vi "testtest.vi"() -> ()   [LabVIEW 2019]
uses:
  <vilib>/WPC Systems Ltd/GECO Driver/Lib/GECOBase/GECO_Driver Class/GECO_SlotName.ctl
  <vilib>/WPC Systems Ltd/GECO Driver/GECODriver/GECO_Initialize_RT/Initialize VIs/Initialize_GECOUnoRT_4HX.vi
  <vilib>/WPC Systems Ltd/GECO Driver/Lib/GECOBase/GECO_Driver Class/Motion/_typedefine/GECO_Motion Operation Mode.ctl
  <vilib>/WPC Systems Ltd/GECO Driver/Lib/GECOBase/GECO_Driver Class/GECO_Driver.lvclass
  <vilib>/WPC Systems Ltd/GECO Driver/Lib/GECOBase/GECO_Driver Class/Motion/_typedefine/GECO_ActiveHighLow.ctl
panel:
  in  "Stop Move":bool
  out "Move Complete?":bool
  out "Logical Position":i32
  out "Encoder Position":i32
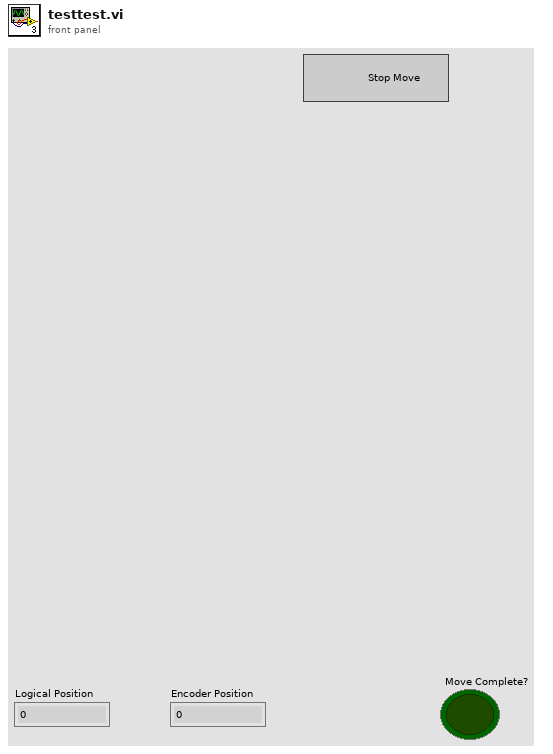
[diagram p1: front panel]
types:
  T1 = typedef "GECO_Driver.lvclass/GECO_SlotName.ctl" = enum16{"C1", "C2", "C3", "C4"}
  T2 = typedef "GECO_Driver.lvclass/GECO_ActiveHighLow.ctl" = enum16{"Active High", "Active Low"}
  T3 = cluster{"Forward Enable":bool, "Forward Polarity":T2}
  T4 = cluster{"Reverse Enable":bool, "Reverse Polarity":T2}
  T5 = typedef "GECO_Driver.lvclass/GECO_Motion Operation Mode.ctl" = enum16{"Absolute Position", "Relative Position", "Velocity"}
  T6 = cluster{"Motion Operation Mode":T5, "Target Position (0)":i32, "Velocity (10000)":i32, "Acceleration (100000)":u32, "Deacceleration (100000)":u32}
  T7 = enum16{"Step/Dir(One Pulse)", "CW/CCW(Two Pulse)"}
  T8 = enum16{"Absolute Position", "Relative Position", "Velocity"}
  T9 = typedef "GECO Motion.lvclass/Axis Select.ctl" = enum16{"Axis 1", "Axis 2", "Axis 3", "Axis 4"}
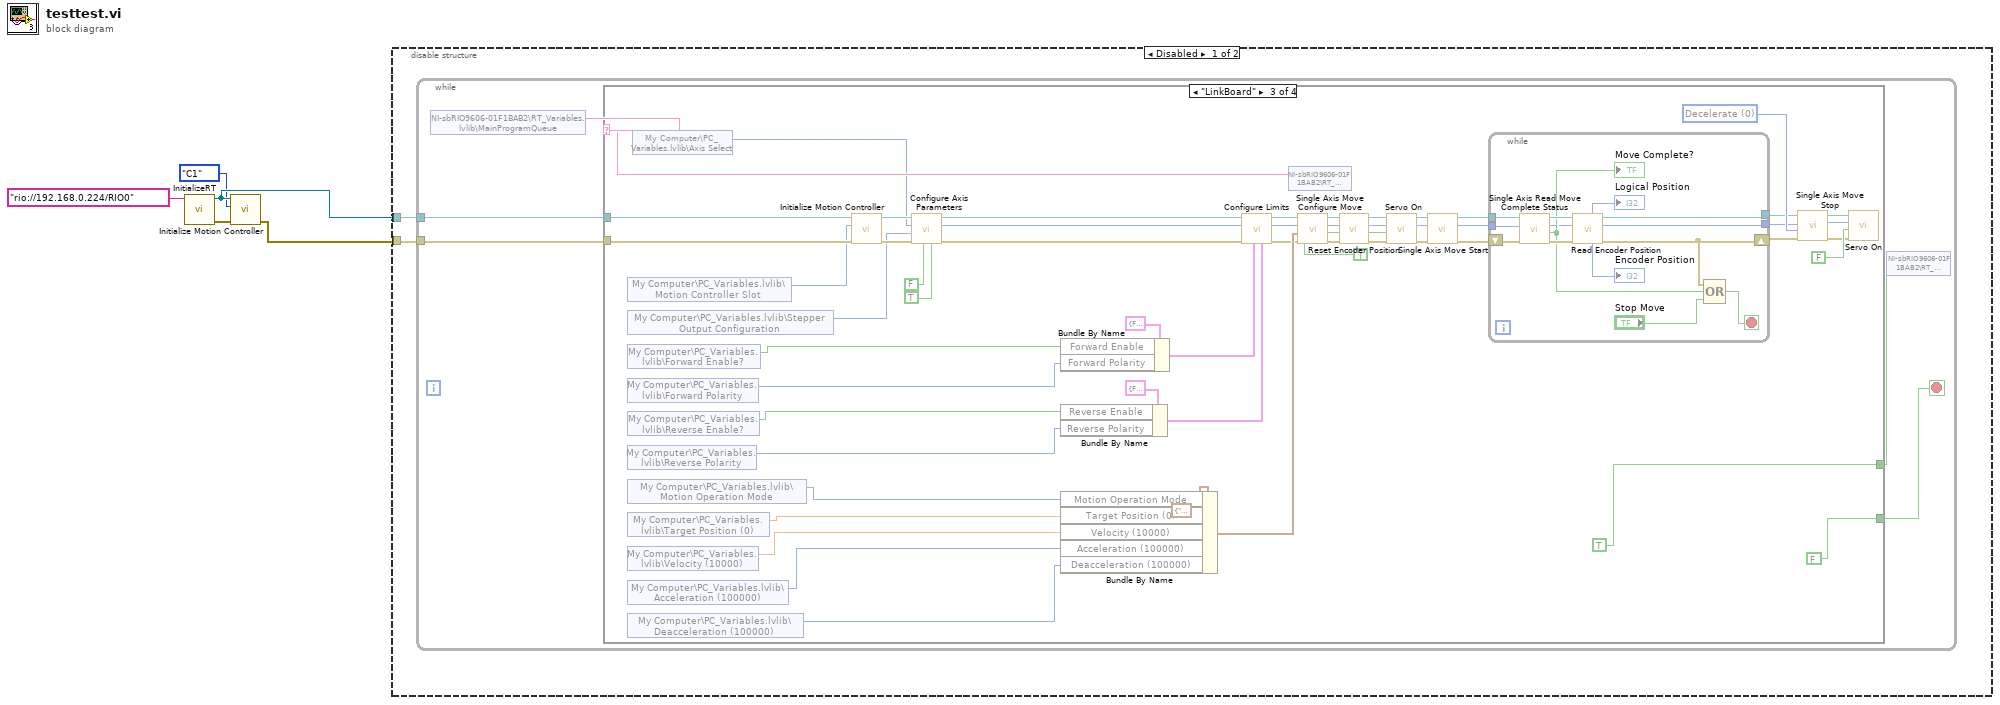
[diagram p0: block diagram]
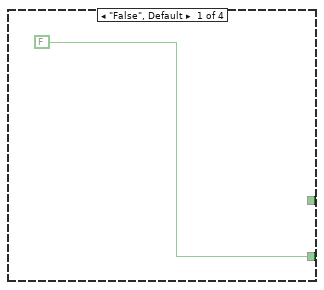
[diagram p2: hidden frame]
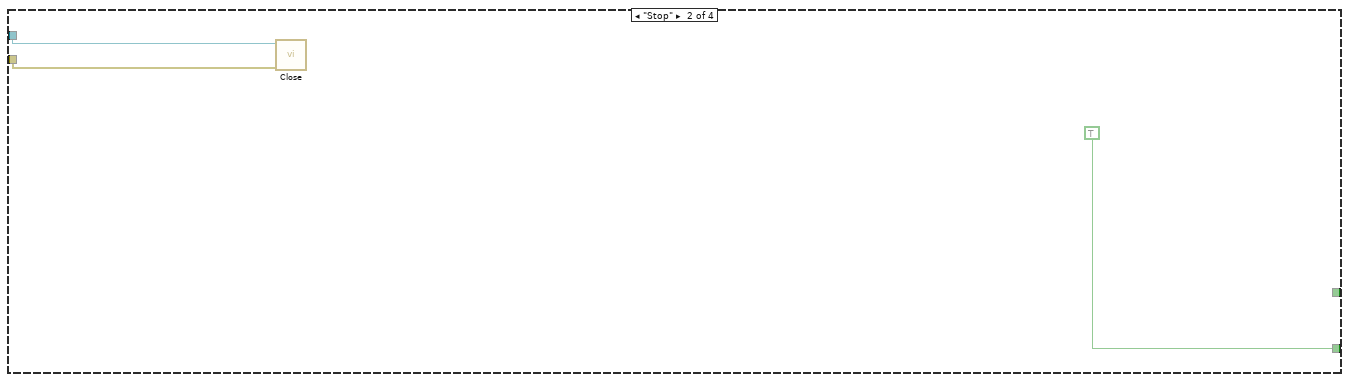
[diagram p3: hidden frame]
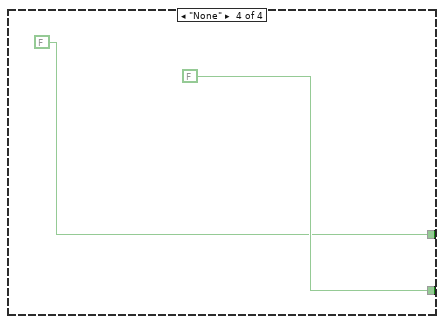
[diagram p4: hidden frame]
diagram:
  n1 = call-poly <vilib>:"InitializeRT.vi"("resource name"=tag "rio://192.168.0.224/RIO0") -> ("error out"=w4:errorcluster, "GECO_Driver out"=w5:refnum<class "GECO_Driver.lvclass">)  [unwired: 9 in]
  n2 = call <vilib>:"Initialize Motion Controller.vi"("error in (no error)"=w4, "Slot"=GECO_SlotName."C1", "GECO_Driver in"=w5) -> ("error out"=w1:errorcluster)  [unwired: 7 in, 1 out]
  n3 = disable-structure shown="Disabled" {
    disable-tunnel: w5 -> [w7 _]
    disable-tunnel: w1 -> [w6 _]
    frame Disabled {
      n4 = while {
        tunnel: w7 -> [w9]
        tunnel: w6 -> [w8]
        stop <- w11 stop-if-true
        n5 = shared-variable "NI-sbRIO9606-01F1BAB2\\RT_Variables.lvlib\\MainProgramQueue"() -> (w12:string)  [unwired: 1 in, 1 out]
        n6 = case shown="\"LinkBoard\"" w12 {
          selector: w12 -> [_ _ w70 _]
          tunnel: [FALSE TRUE FALSE FALSE] -> w11
          tunnel: [_ _ TRUE FALSE] -> w10
          tunnel: w9 -> [_ w14 w38 _]
          tunnel: w8 -> [_ w15 w37 _]
          frame "False", Default {
          }
          frame "Stop" {
            n7 = call <vilib>:"Close.vi"("error in (no error)"=w15, "GECO_Driver in"=w14) -> ()  [unwired: 9 in, 1 out]
          }
          frame "LinkBoard" {
            w36 = u16 0 items=["Decelerate", "Halt"] ("Motion Stop Type")
            n8 = shared-variable "My Computer\\PC_Variables.lvlib\\Motion Controller Slot"() -> (w26:enum16{"C1", "C2", "C3", "C4"})  [unwired: 1 in, 1 out]
            n9 = shared-variable "My Computer\\PC_Variables.lvlib\\Stepper Output Configuration"() -> (w27:T7)  [unwired: 1 in, 1 out]
            n10 = shared-variable "My Computer\\PC_Variables.lvlib\\Forward Enable?"() -> (w25:bool)  [unwired: 1 in, 1 out]
            n11 = shared-variable "My Computer\\PC_Variables.lvlib\\Forward Polarity"() -> (w24:enum16{"Active High", "Active Low"})  [unwired: 1 in, 1 out]
            n12 = shared-variable "My Computer\\PC_Variables.lvlib\\Reverse Enable?"() -> (w23:bool)  [unwired: 1 in, 1 out]
            n13 = shared-variable "My Computer\\PC_Variables.lvlib\\Reverse Polarity"() -> (w22:enum16{"Active High", "Active Low"})  [unwired: 1 in, 1 out]
            n14 = shared-variable "My Computer\\PC_Variables.lvlib\\Motion Operation Mode"() -> (w21:T8)  [unwired: 1 in, 1 out]
            n15 = shared-variable "My Computer\\PC_Variables.lvlib\\Target Position (0)"() -> (w20:dbl)  [unwired: 1 in, 1 out]
            n16 = shared-variable "My Computer\\PC_Variables.lvlib\\Velocity (10000)"() -> (w19:dbl)  [unwired: 1 in, 1 out]
            n17 = shared-variable "My Computer\\PC_Variables.lvlib\\Acceleration (100000)"() -> (w18:u32)  [unwired: 1 in, 1 out]
            n18 = shared-variable "My Computer\\PC_Variables.lvlib\\Deacceleration (100000)"() -> (w17:u32)  [unwired: 1 in, 1 out]
            n19 = shared-variable "My Computer\\PC_Variables.lvlib\\Axis Select"() -> (w28:enum16{"Axis 1", "Axis 2", "Axis 3", "Axis 4"})  [unwired: 1 in, 1 out]
            n20 = call <vilib>:"Initialize Motion Controller.vi"("error in (no error)"=w37, "Slot"=w26, "GECO_Driver in"=w38) -> ("error out"=w59:errorcluster, "Motion reference out"=w58:refnum<class "GECO Motion.lvclass">)  [unwired: 7 in]
            n21 = call <vilib>:"Configure Axis Parameters.vi"("Reverse Encoder Direction?"=TRUE ("Encoder Direction"), "Reverse Axis Direction?"=FALSE ("Axis Direction"), "error in (no error)"=w59, "Stepper Output Configuration"=w27, "Axis Select"=w28, "GECO Motion in"=w58) -> ("error out"=w52:errorcluster, "Axis Select out"=w62:T9, "GECO Motion out"=w51:refnum<class "GECO Motion.lvclass">)  [unwired: 3 in]
            n22 = Bundle By Name(cluster=T3 {"Forward Enable"=FALSE, "Forward Polarity"=enum."Active Low"} ("Forward"), "Forward Enable"=w25, "Forward Polarity"=w24) -> (w60:T3)
            n23 = Bundle By Name(cluster=T4 {"Reverse Enable"=FALSE, "Reverse Polarity"=enum."Active Low"} ("Reverse"), "Reverse Enable"=w23, "Reverse Polarity"=w22) -> (w61:T4)
            n24 = Bundle By Name(cluster=T6 {"Motion Operation Mode"=enum."Absolute Position", "Target Position (0)"=0, "Velocity (10000)"=10000, "Acceleration (100000)"=100000, "Deacceleration (100000)"=100000} ("Singel Axis Move Paramters"), "Motion Operation Mode"=w21, "Target Position (0)"=w20, "Velocity (10000)"=w19, "Acceleration (100000)"=w18, "Deacceleration (100000)"=w17) -> (w57:T6)
            n25 = call <vilib>:"Configure Limits.vi"("Reverse"=w61, "Forward"=w60, "error in (no error)"=w52, "Axis Select"=w62, "GECO Motion in"=w51) -> ("error out"=w54:errorcluster, "Axis Select out"=w63:T9, "GECO Motion out"=w53:refnum<class "GECO Motion.lvclass">)  [unwired: 4 in]
            n26 = shared-variable "NI-sbRIO9606-01F1BAB2\\RT_Variables.lvlib\\text"(w70) -> ()  [unwired: 1 in, 1 out]
            n27 = call <vilib>:"Single Axis Move Configure Move.vi"("error in (no error)"=w54, "Singel Axis Move Paramters"=w57, "Axis Select"=w63, "GECO Motion in"=w53) -> ("error out"=w56:errorcluster, "Axis Select out"=w64:T9, "GECO Motion out"=w55:refnum<class "GECO Motion.lvclass">)  [unwired: 5 in]
            n28 = call <vilib>:"Reset Encoder Position.vi"("error in (no error)"=w56, "Axis Select"=w64, "GECO Motion in"=w55) -> ("error out"=w50:errorcluster, "Axis Select out"=w65:T9, "GECO Motion out"=w49:refnum<class "GECO Motion.lvclass">)  [unwired: 6 in]
            n29 = call <vilib>:"Servo On.vi"("error in (no error)"=w50, "Servo On"=TRUE, "Axis Select"=w65, "GECO Motion in"=w49) -> ("error out"=w46:errorcluster, "Axis Select out"=w66:T9, "GECO Motion out"=w45:refnum<class "GECO Motion.lvclass">)  [unwired: 5 in]
            n30 = call <vilib>:"Single Axis Move Start.vi"("error in (no error)"=w46, "Axis Select"=w66, "GECO Motion in"=w45) -> ("error out"=w48:errorcluster, "Axis Select out"=w67:T9, "GECO Motion out"=w47:refnum<class "GECO Motion.lvclass">)  [unwired: 6 in]
            n31 = while {
              tunnel: w47 -> [w77]
              tunnel: [w82] -> w31
              shift-right: [w79] -> w30
              shift-left: w48 -> [w78]
              tunnel: w67 -> [w73]
              tunnel: [w71] -> w29
              stop <- w83 stop-if-true
              n32 = call <vilib>:"Single Axis Read Move Complete Status.vi"("error in (no error)"=w78, "Axis Select"=w73, "GECO Motion in"=w77) -> ("error out"=w80:errorcluster, "Move Complete?"=w76:bool, "Axis Select out"=w72:T9, "GECO Motion out"=w81:refnum<class "GECO Motion.lvclass">)  [unwired: 5 in]
              "Move Complete?" <- w76
              n33 = call <vilib>:"Read Encoder Position.vi"("error in (no error)"=w80, "Axis Select"=w72, "GECO Motion in"=w81) -> ("error out"=w79:errorcluster, "Axis Select out"=w71:T9, "GECO Motion out"=w82:refnum<class "GECO Motion.lvclass">, "Encoder Position"=→"Encoder Position":i32, "Logical Position"=→"Logical Position":i32)  [unwired: 4 in]
              n34 = Compound Arithmetic op=OR(w79, w76, "Stop Move") -> (w83:bool)
            }
            n35 = call <vilib>:"Single Axis Move Stop.vi"("error in (no error)"=w30, "Motion Stop Type"=w36, "Axis Select"=w29, "GECO Motion in"=w31) -> ("error out"=w33:errorcluster, "Axis Select out"=w32:T9, "GECO Motion out"=w34:refnum<class "GECO Motion.lvclass">)  [unwired: 5 in]
            n36 = call <vilib>:"Servo On.vi"("error in (no error)"=w33, "Servo On"=FALSE, "Axis Select"=w32, "GECO Motion in"=w34) -> ()  [unwired: 5 in, 3 out]
          }
          frame "None" {
          }
        }
        n37 = shared-variable "NI-sbRIO9606-01F1BAB2\\RT_Variables.lvlib\\LED"(w10) -> ()  [unwired: 1 in, 1 out]
      }
    }
    frame Enabled {
    }
  }
